vi "para.vi"(6 "Reset":bool) -> (2 "Parametr J":dbl, 3 "czas cyklu":dbl)   [LabVIEW 2025]
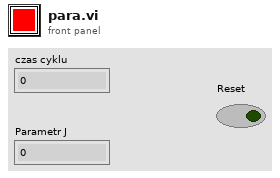
[diagram p1: front panel]
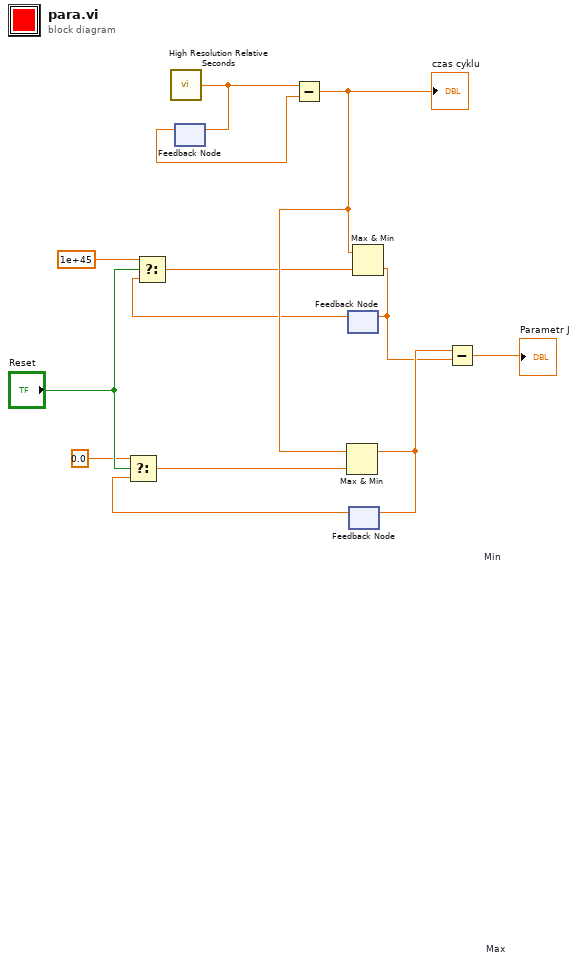
[diagram p0: block diagram]
diagram:
  n1 = call <vilib>:"High Resolution Relative Seconds.vi"() -> ("relative seconds"=w13:dbl)
  n2 = feedback-in #1(w13) -> ()
  n3 = feedback #1() -> (w12:dbl)  [unwired: 1 in]
  n4 = Subtract(x=w13, y=w12) -> (x-y=w11:dbl)
  "czas cyklu" <- w11
  n5 = feedback #2 "Min"() -> (w2:dbl)  [unwired: 1 in]
  n6 = Select(t=1e+45, s="Reset", f=w2) -> (s? t:f=w1:dbl)
  n7 = feedback #3 "Max"() -> (w4:dbl)  [unwired: 1 in]
  n8 = Select(t=0.0, s="Reset", f=w4) -> (s? t:f=w3:dbl)
  n9 = Max & Min(x=w11, y=w3) -> (max(x,y)=w10:dbl)  [unwired: 1 out]
  n10 = feedback-in #3(w10) -> ()
  n11 = Max & Min(x=w11, y=w1) -> (min(x,y)=w9:dbl)  [unwired: 1 out]
  n12 = feedback-in #2(w9) -> ()
  n13 = Subtract(x=w10, y=w9) -> (x-y=→"Parametr J":dbl)
